vi "XML.InsertChildTextNode.vi"(7 "parent":u32, 8 "error in":errorcluster, 9 "text":string, 10 "name":string, 11 "doc":u32) -> (0 "error out":errorcluster, 3 "doc out":u32)   [LabVIEW 2019, in "Tools.lvlib"]
uses:
  Tools.lvlib
  LibXML/LibXML.lvlib
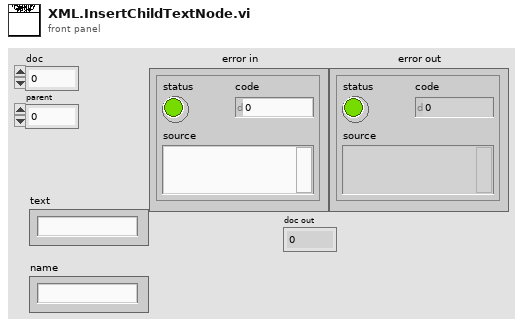
[diagram p1: front panel]
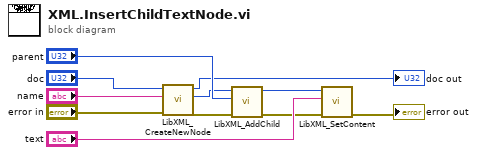
[diagram p0: block diagram]
diagram:
  n1 = call "LibXML_CreateNewNode.vi"("error in"="error in", "name"="name", "doc"="doc") -> ("error out"=w6:errorcluster, "nodePtr out"=w1:u32, "doc out"=→"doc out":u32)  [unwired: 6 in]
  n2 = call "LibXML_AddChild.vi"("error in"=w6, "parent"="parent", "node"=w1) -> ("error out"=w5:errorcluster, "node copy"=w7:u32)  [unwired: 7 in]
  n3 = call "LibXML_SetContent.vi"("error in (no error)"=w5, "content"="text", "node"=w7) -> ("error out"=→"error out":errorcluster)  [unwired: 7 in, 1 out]
